vi "VIE.Module.Queued Message Handler.enqueue.State.PolyChild.QueuedMessageHandler.vi"(6 "Where to Enque (End of the Queue)":enum16{"Start of the Queue", "End of the Queue"}(ring)=enum."End of the Queue", 8 "error in (no error)":errorcluster, 9 "State to Enqueue":string, 10 "QueuedMessageHandler.dqGOOPClass (in)":T1) -> (0 "error out":errorcluster, 2 "QueuedMessageHandler.dqGOOPClass (out)":T1)   [LabVIEW 2010, in "VIE.Module.Queued Message Handler.QueuedMessageHandler.dqGOOPClass.lvlib"]
uses:
  VIE.Module.Queued Message Handler.QueuedMessageHandler.dqGOOPClass.lvlib
  VIE.Module.Queued Message Handler.dqClass_ObjectReference.ctl
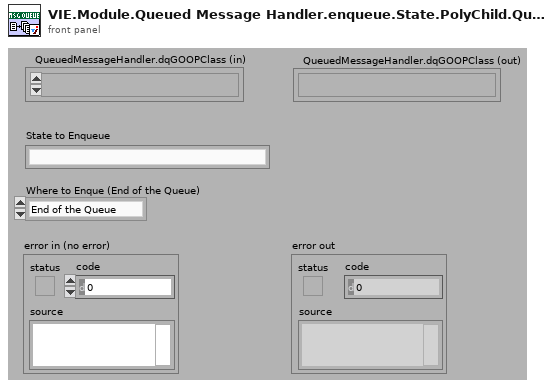
[diagram p1: front panel]
types:
  T1 = typedef "VIE.Module.Queued Message Handler.QueuedMessageHandler.dqGOOPClass.lvlib/VIE.Module.Queued Message Handler.dqClass_ObjectReference.ctl" = refnum<k1>
  T2 = typedef "VIE.Module.Queued Message Handler.QueuedMessageHandler.dqGOOPClass.lvlib/VIE.Module.Queued Message Handler.dqClass_ObjectData.ctl" = cluster{"Message Queue":refnum<queue>, "Log File Refnum":refnum<file>}
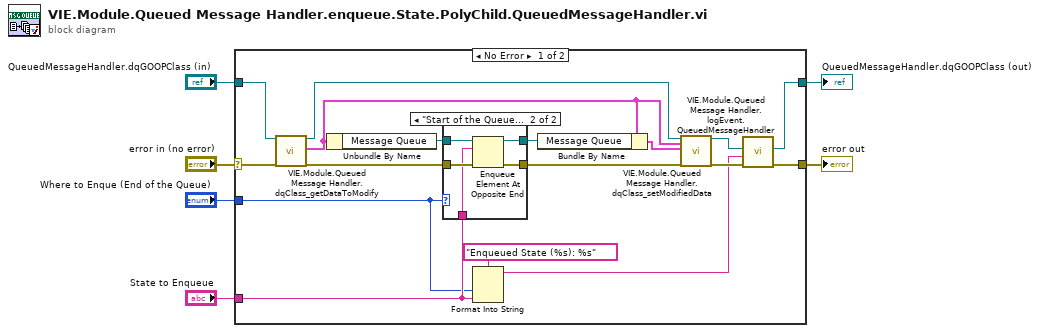
[diagram p0: block diagram]
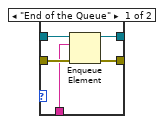
[diagram p2: hidden frame]
diagram:
  n1 = case shown="No Error" "error in (no error)" {
    selector: "error in (no error)" -> [w20 w35]
    tunnel: [w9 w35] -> w5
    tunnel: [w10 w34] -> w4
    tunnel: "QueuedMessageHandler.dqGOOPClass (in)" -> [w18 w34]
    tunnel: "State to Enqueue" -> [w8 _]
    tunnel: "Where to Enque (End of the Queue)" -> [w7 _]
    frame No Error {
      n2 = call "VIE.Module.Queued Message Handler.dqClass_getDataToModify.vi"("reference"=w18, "error in (no error)"=w20) -> ("duplicate reference"=w14:T1, "data"=w15:T2, "error out"=w19:errorcluster)  [unwired: 14 in, 1 out]
      n3 = Unbundle By Name(w15) -> ("Message Queue"=w23:refnum<queue>)
      n4 = case shown="\"Start of the Queue\"" w7 {
        tunnel: w23 -> [w28 w33]
        tunnel: [w27 w32] -> w22
        tunnel: w19 -> [w26 w31]
        tunnel: [w25 w30] -> w17
        tunnel: w8 -> [w24 w29]
        frame "End of the Queue" {
          n5 = Enqueue Element(queue=w28, element=w24, error in (no error)=w26) -> (queue out=w27:refnum<queue>, error out=w25:errorcluster)  [unwired: 1 in, 1 out]
        }
        frame "Start of the Queue" {
          n6 = Enqueue Element At Opposite End(queue=w33, element=w29, error in (no error)=w31) -> (queue out=w32:refnum<queue>, error out=w30:errorcluster)  [unwired: 1 in, 1 out]
        }
      }
      n7 = Format Into String(format string="Enqueued State (%s): %s", w7, w8) -> (resulting string=w12:string)  [unwired: 2 in, 1 out]
      n8 = Bundle By Name(cluster=w15, "Message Queue"=w22) -> (w16:T2)
      n9 = call "VIE.Module.Queued Message Handler.dqClass_setModifiedData.vi"("reference"=w14, "data (unmodified)"=w15, "data"=w16, "error in (no error)"=w17) -> ("duplicate reference"=w11:T1, "error out"=w13:errorcluster)  [unwired: 14 in]
      n10 = call "VIE.Module.Queued Message Handler.logEvent.QueuedMessageHandler.vi"("error in (no error)"=w13, "Event to Log"=w12, "QueuedMessageHandler.dqGOOPClass (in)"=w11) -> ("error out"=w9:errorcluster, "QueuedMessageHandler.dqGOOPClass (out)"=w10:T1)  [unwired: 7 in]
    }
    frame Error {
    }
  }
  "error out" <- w5
  "QueuedMessageHandler.dqGOOPClass (out)" <- w4
